vi "parse_error_code.vi"(10 "source":string, 11 "code":i32) -> (3 "parsed_error_string":string)   [LabVIEW 2020]
uses:
  <vilib>/Utility/error.llb/DialogType.ctl
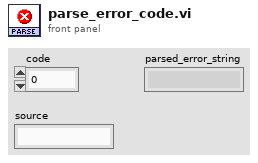
[diagram p1: front panel]
types:
  T1 = typedef "DialogType.ctl" = u16
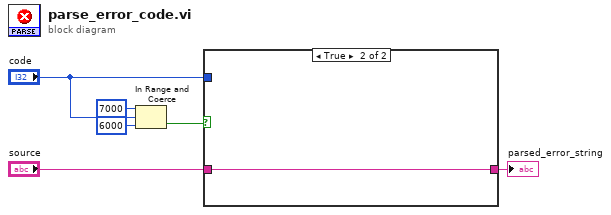
[diagram p0: block diagram]
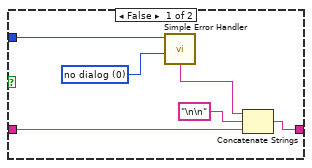
[diagram p2: hidden frame]
diagram:
  n1 = In Range and Coerce(upper limit=7000, x="code", lower limit=6000) -> (In Range?=w4:bool)  [unwired: 1 out]
  n2 = case shown="True" w4 {
    tunnel: "source" -> [w11 w13]
    tunnel: [w9 w13] -> w5
    tunnel: "code" -> [w7 _]
    frame False {
      w8 = T1 0 items=["no dialog", "OK message", "continue or stop message", "OK message + warnings", "continue/stop + warnings"] ("type of dialog (OK msg:1)")
      n3 = call <vilib>:"Simple Error Handler.vi"("error code (no error:0)"=w7, "type of dialog (OK msg:1)"=w8) -> ("message"=w12:string)  [unwired: 3 in, 4 out]
      n4 = Concatenate Strings(w12, "\n\n" ("element"), w11) -> (w9:string)
    }
    frame True {
    }
  }
  "parsed_error_string" <- w5
